vi "Load Subsystem IO Logging Attributes.vi"(7 "Headers":string[](array[string]), 8 "error in (no error)":errorcluster, 10 "Raw Configuration":string[](array[string]), 11 "Subsystem I/O Attributes In":T1={"Name"="", "Data Type"=enum."double", "Access Type"=enum."Read only", "Alarm Enabled?"=FALSE, "Logging Enabled?"=FALSE, "Logging Attributes"={"log data? (F)"=TRUE, "log alarms & events? (F)"=TRUE}, "Alarm Attributes"={"Hi:enable? (F)"=TRUE, "Hi:name"="Hi Alarm Test", "Hi:level/change"=1.0, "Lo:enable? (F)"=TRUE, "Lo:name"="Lo", "Lo:level/change"=25.0, "Boolean:enable? (F)"=TRUE, "Boolean:name"="Boolean", "Boolean:value"=TRUE, "BadStatus:enable? (F)"=TRUE, "BadStatus:name"="BadStatus"}}) -> (0 "error out":errorcluster, 2 "dup Raw Configuration":string[](array[string]), 3 "Subsystem I/O Item Attributes Out":T1={"Name"="", "Data Type"=enum."double", "Access Type"=enum."Read only", "Alarm Enabled?"=FALSE, "Logging Enabled?"=FALSE, "Logging Attributes"={"log data? (F)"=TRUE, "log alarms & events? (F)"=TRUE}, "Alarm Attributes"={"Hi:enable? (F)"=TRUE, "Hi:name"="Hi Alarm Test", "Hi:level/change"=1.0, "Lo:enable? (F)"=TRUE, "Lo:name"="Lo", "Lo:level/change"=25.0, "Boolean:enable? (F)"=TRUE, "Boolean:name"="Boolean", "Boolean:value"=TRUE, "BadStatus:enable? (F)"=TRUE, "BadStatus:name"="BadStatus"}})   [LabVIEW 2024]
doc: "Loads logging attributes."
uses:
  Controls/Server/Subsystem IO Attributes.ctl
  Controls/Server/Subsystem IO Logging Attributes.ctl
  Controls/Server/Subsystem IO Alarm Attributes.ctl
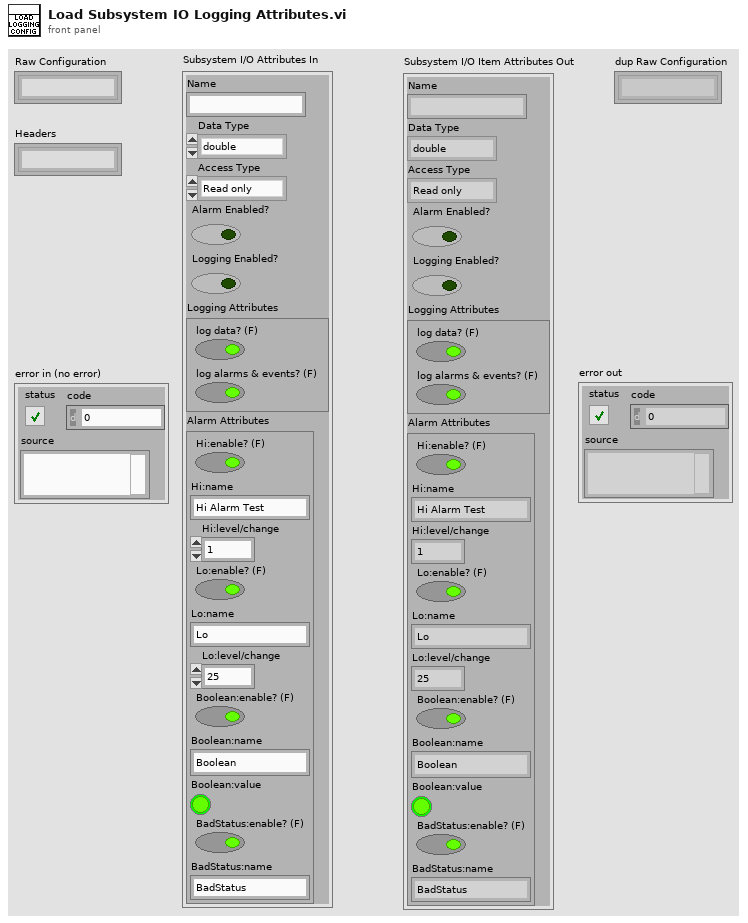
[diagram p1: front panel]
types:
  T1 = typedef "Subsystem IO Attributes.ctl" = cluster{"Name":string, "Data Type":enum32{"u32BitField", "bool", "double", "string", "int8", "uint8", "int16", "uint16", "int32", "uint32", "int64", "uint64", "single", "double waveform", "int16 waveform", "array of boolean", "array of int8", "array of uint8", "array of int16", "array of uint16", "array of int32", "array of uint32", "array of int64", "array of uint64", "array of single", "array of double", "array of double waveform", "array of int16 waveform", "array of string", "variant", "timestamp", "fixed point", "custom"}, "Access Type":enum32{"Read only", "Write only", "Read/write"}, "Alarm Enabled?":bool, "Logging Enabled?":bool, "Logging Attributes":T2, "Alarm Attributes":T3}
  T2 = typedef "Subsystem IO Logging Attributes.ctl" = cluster{"log data? (F)":bool, "log alarms & events? (F)":bool}
  T3 = typedef "Subsystem IO Alarm Attributes.ctl" = cluster{"Hi:enable? (F)":bool, "Hi:name":string, "Hi:level/change":dbl, "Lo:enable? (F)":bool, "Lo:name":string, "Lo:level/change":dbl, "Boolean:enable? (F)":bool, "Boolean:name":string, "Boolean:value":bool, "BadStatus:enable? (F)":bool, "BadStatus:name":string}
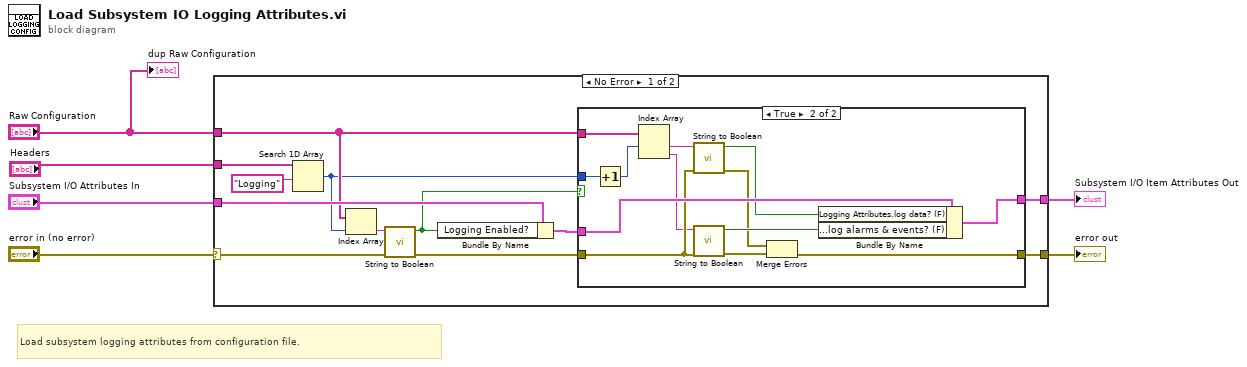
[diagram p0: block diagram]
diagram:
  # "Load subsystem logging attributes from configuration file."
  n1 = case shown="No Error" "error in (no error)" {
    selector: "error in (no error)" -> [w17 w35]
    tunnel: [w13 w35] -> w5
    tunnel: "Subsystem I/O Attributes In" -> [w12 w34]
    tunnel: [w15 w34] -> w3
    tunnel: "Raw Configuration" -> [w10 _]
    tunnel: "Headers" -> [w7 _]
    frame No Error {
      n2 = Search 1D Array(1D array=w7, element="Logging") -> (index of element=w8:i32)  [unwired: 1 in]
      n3 = Index Array(array=w10, index=w8) -> (element=w18:string)
      n4 = call "String to Boolean.vi"("error in (no error)"=w17, "Boolean String"=w18) -> ("error out"=w14:errorcluster, "Boolean"=w11:bool)  [unwired: 8 in]
      n5 = Bundle By Name(cluster=w12, "Logging Enabled?"=w11) -> (w16:T1)
      n6 = case shown="True" w11 {
        tunnel: w16 -> [w20 w33]
        tunnel: [w20 w32] -> w15
        tunnel: w14 -> [w19 w28]
        tunnel: [w19 w22] -> w13
        tunnel: w10 -> [_ w31]
        tunnel: w8 -> [_ w30]
        frame False {
        }
        frame True {
          n7 = Increment(x=w30) -> (x+1=w29:i32)
          n8 = Index Array(array=w31, index #1=w29) -> (element #1=w26:string, element #2=w27:string)  [unwired: 1 in]
          n9 = call "String to Boolean.vi"("error in (no error)"=w28, "Boolean String"=w26) -> ("error out"=w21:errorcluster, "Boolean"=w25:bool)  [unwired: 8 in]
          n10 = call "String to Boolean.vi"("error in (no error)"=w28, "Boolean String"=w27) -> ("error out"=w23:errorcluster, "Boolean"=w24:bool)  [unwired: 8 in]
          n11 = Merge Errors(w21, w23) -> (w22:errorcluster)
          n12 = Bundle By Name(cluster=w33, "Logging Attributes.log data? (F)"=w25, "Logging Attributes.log alarms & events? (F)"=w24) -> (w32:T1)
        }
      }
    }
    frame Error {
    }
  }
  "error out" <- w5
  "Subsystem I/O Item Attributes Out" <- w3
  "dup Raw Configuration" <- "Raw Configuration"
